vi "Load Sequences.vi"(5 "Byte 2 Ch.":u8[](array[numeric]), 6 "Byte 3 Timing Delay":u8[](array[numeric]), 7 "Byte 1 Ch.":u8[](array[numeric]), 8 "error in (no error)":errorcluster, 11 "VISA resource name":refnum<visa-resource-name>) -> (0 "error out":errorcluster, 3 "VISA resource name out":refnum<visa-resource-name>)   [LabVIEW 2020, in "QuPMXdriver.lvlib"]
doc: "Loads sequences represented as bytes into multiplexer."
uses:
  QuPMXdriver.lvlib
  <vilib>/Utility/error.llb/Error Cluster From Error Code.vi
  <vilib>/ErrorRing/Error Ring.xnode
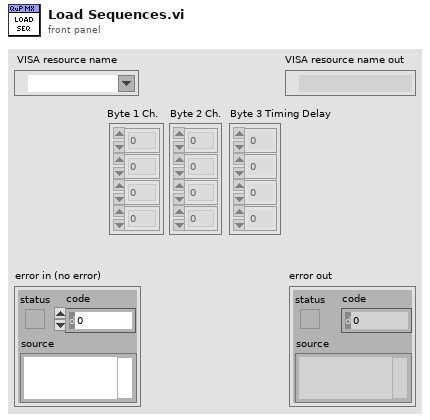
[diagram p1: front panel]
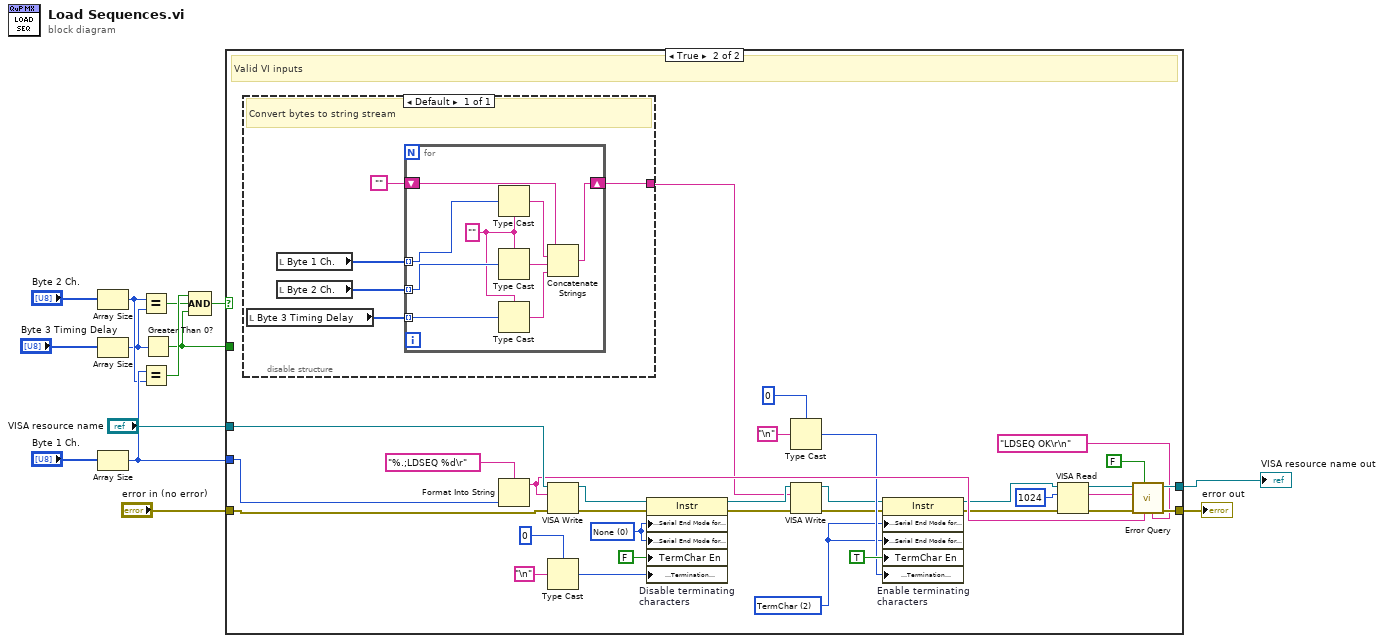
[diagram p0: block diagram]
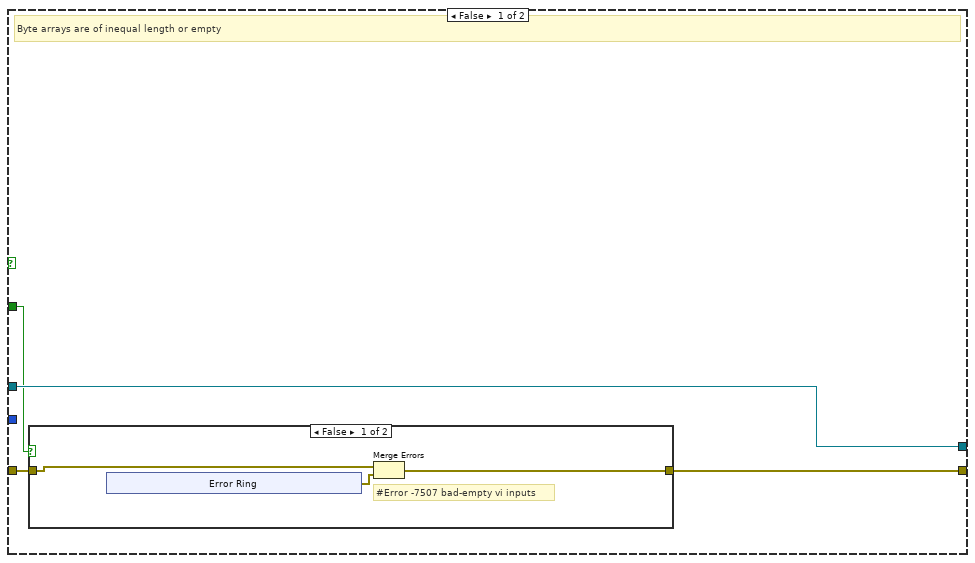
[diagram p2: hidden frame]
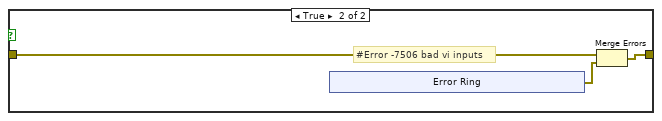
[diagram p3: hidden frame]
diagram:
  n1 = Array Size(array="Byte 2 Ch.") -> (size(s)=w5:i32)
  n2 = Array Size(array="Byte 3 Timing Delay") -> (size(s)=w2:i32)
  n3 = Array Size(array="Byte 1 Ch.") -> (size(s)=w6:i32)
  n4 = Equal?(x=w5, y=w2) -> (x = y?=w4:bool)
  n5 = Equal?(x=w6, y=w5) -> (x = y?=w7:bool)
  n6 = Greater Than 0?(x=w2) -> (x > 0?=w1:bool)
  n7 = Compound Arithmetic op=AND(w7, w4, w1) -> (w3:bool)
  n8 = case shown="True" w3 {
    tunnel: "VISA resource name" -> [w18 w66]
    tunnel: "error in (no error)" -> [w15 w65]
    tunnel: [w16 w63] -> w12
    tunnel: [w18 w62] -> w11
    tunnel: w6 -> [_ w40]
    tunnel: w1 -> [w17 _]
    frame False {
      # "Byte arrays are of inequal length or empty"
      n9 = case shown="False" w17 {
        tunnel: w15 -> [w20 w29]
        tunnel: [w19 w27] -> w16
        frame False {
          # "#Error -7507 bad-empty vi inputs"
          n10 = xnode "Error Ring"() -> ("error out"=w21:errorcluster)
          n11 = Merge Errors(w20, w21) -> (w19:errorcluster)
        }
        frame True {
          # "#Error -7506 bad vi inputs"
          n12 = xnode "Error Ring"() -> ("error out"=w28:errorcluster)
          n13 = Merge Errors(w29, w28) -> (w27:errorcluster)
        }
      }
    }
    frame True {
      w47 = u16 2 items=["None", "LastBit", "TermChar"] ("Serial Settings:Serial End Mode for Reads")
      w52 = u16 0 items=["None", "LastBit", "TermChar"] ("Serial Settings:Serial End Mode for Reads")
      # "Valid VI inputs"
      n14 = disable-structure shown="Default" {
        disable-tunnel: [w67] -> w37
        frame Enabled {
          # "Convert bytes to string stream"
          n15 = local read "Byte 3 Timing Delay"() -> (w69:u8[])
          n16 = local read "Byte 1 Ch."() -> (w71:u8[])
          n17 = local read "Byte 2 Ch."() -> (w70:u8[])
          n18 = for {
            tunnel: w71 -> [w80] mode=indexing
            tunnel: w70 -> [w79] mode=indexing
            tunnel: w69 -> [w78] mode=indexing
            shift-right: [w74] -> w67
            shift-left: "" -> [w73]
            w72 = "" ("type")
            n19 = Type Cast(type=w72, x=w80) -> (*(type *) &x=w76:string)
            n20 = Type Cast(type=w72, x=w79) -> (*(type *) &x=w77:string)
            n21 = Type Cast(type=w72, x=w78) -> (*(type *) &x=w75:string)
            n22 = Concatenate Strings(w73, w76, w77, w75) -> (w74:string)
          }
        }
      }
      n23 = Format Into String(format string="%.;LDSEQ %d\r" ("write buffer"), w40) -> (resulting string=w55:string)  [unwired: 2 in, 1 out]
      n24 = VISA Write(VISA resource name=w66, write buffer=w55, error in (no error)=w65) -> (VISA resource name out=w44:refnum<visa-resource-name>, error out=w43:errorcluster)  [unwired: 1 out]
      n25 = Type Cast(type=u8 0, x="\n" ("Line Feed Constant")) -> (*(type *) &x=w53:u8)
      n26 = property on="Disable terminating\ncharacters" class="Instr"(reference=w44, error in=w43, "Serial Settings:Serial End Mode for Reads"=w52, "Serial Settings:Serial End Mode for Writes"=w52, "TermChar En"=FALSE ("Message Based Settings:Termination Character Enable"), "Message Based Settings:Termination Character"=w53) -> (reference out=w38:refnum<visa-resource-name>, error out=w39:errorcluster)
      n27 = Type Cast(type=u8 0, x="\n" ("Line Feed Constant")) -> (*(type *) &x=w48:u8)
      n28 = VISA Write(VISA resource name=w38, write buffer=w37, error in (no error)=w39) -> (VISA resource name out=w36:refnum<visa-resource-name>, error out=w35:errorcluster)  [unwired: 1 out]
      n29 = property on="Enable terminating\ncharacters" class="Instr"(reference=w36, error in=w35, "Serial Settings:Serial End Mode for Reads"=w47, "Serial Settings:Serial End Mode for Writes"=w47, "TermChar En"=TRUE ("Message Based Settings:Termination Character Enable"), "Message Based Settings:Termination Character"=w48) -> (reference out=w42:refnum<visa-resource-name>, error out=w41:errorcluster)
      n30 = VISA Read(VISA resource name=w42, byte count=u32 1024, error in (no error)=w41) -> (VISA resource name out=w59:refnum<visa-resource-name>, read buffer=w57:string, error out=w58:errorcluster)  [unwired: 1 out]
      n31 = call "Error Query.vi"("Expected read buffer"="LDSEQ OK\r\n", "Last command"=w55, "Ignore empty sequence? (T)"=FALSE, "error in (no error)"=w58, "Read buffer"=w57, "VISA resource name"=w59) -> ("error out"=w63:errorcluster, "VISA resource name out"=w62:refnum<visa-resource-name>)  [unwired: 4 in]
    }
  }
  "error out" <- w12
  "VISA resource name out" <- w11
